vi "Assisstant Reply.vi"(8 "error in (no error)":errorcluster, 10 "assisstant_response":refnum<class "abstract_message_base.lvclass">, 11 "simple_html_chat_ui in":refnum<class "simple_html_chat_ui.lvclass">) -> (0 "error out":errorcluster, 3 "simple_html_chat_ui out":refnum<class "simple_html_chat_ui.lvclass">)   [LabVIEW 2020, in "simple_html_chat_ui.lvclass"]
doc: "To writer the assisstant response to the html page through the websocket"
uses:
  simple_html_chat_ui.lvclass
  models/abstract_message_base/abstract_message_base.lvclass
  models/message_text/message_text.lvclass
  dependencies/WebSockets-API/Source/WebSockets/WebSocket Server/WebSocket Server.lvclass
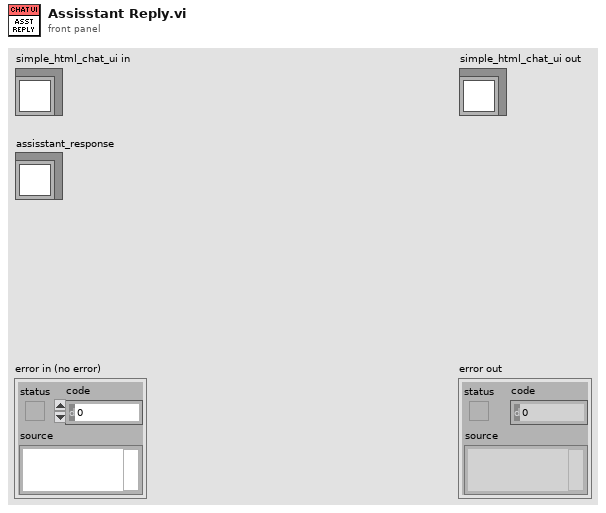
[diagram p1: front panel]
types:
  T1 = typedef "message_text.lvclass/message.ctl" = cluster{"role":string, "content":string[]}
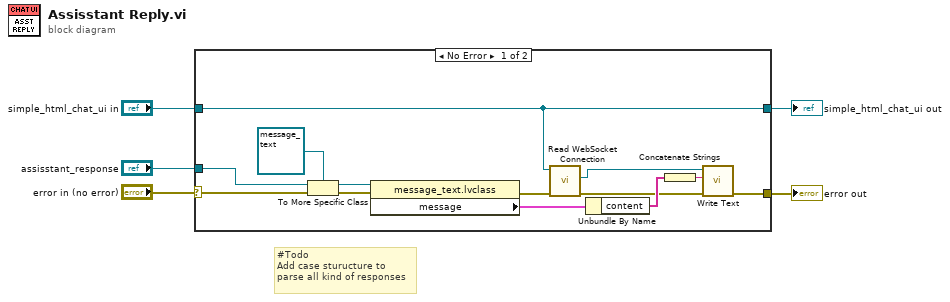
[diagram p0: block diagram]
diagram:
  # "#Todo \nAdd case sturucture to\nparse all kind of responses"
  n1 = case shown="No Error" "error in (no error)" {
    selector: "error in (no error)" -> [w17 w20]
    tunnel: [w16 w20] -> w4
    tunnel: [w6 w19] -> w2
    tunnel: "simple_html_chat_ui in" -> [w6 w19]
    tunnel: "assisstant_response" -> [w18 _]
    frame No Error {
      n2 = To More Specific Class(target class=refnum<class "message_text.lvclass"> refnum ("message_text.lvclass"), reference=w18, error in=w17) -> (specific class reference=w8:refnum<class "message_text.lvclass">, error out=w7:errorcluster)
      n3 = property class="message_text.lvclass"(reference=w8, error in=w7) -> (error out=w12:errorcluster, "message"=w15:T1)  [unwired: 1 out]
      n4 = call-dynamic "Read WebSocket Connection.vi"("error in (no error)"=w12, "simple_html_chat_ui in"=w6) -> ("error out"=w11:errorcluster, "WebSockets.lvlib:WebSocket Server"=w10:refnum<class "WebSocket Server.lvclass">)  [unwired: 7 in, 1 out]
      n5 = Unbundle By Name(w15) -> ("content"=w14:string[])
      n6 = Concatenate Strings(w14) -> (w13:string)
      n7 = call-dynamic "Write Text.vi"("error in (no error)"=w11, "String Data"=w13, "WebSocket in"=w10) -> ("error out"=w16:errorcluster)  [unwired: 7 in, 1 out]
    }
    frame Error {
    }
  }
  "error out" <- w4
  "simple_html_chat_ui out" <- w2
